vi "LaserExample.vi"() -> ()   [LabVIEW 2015]
panel:
  out "OK (Only RX Commands)":bool
  out "command received":bool
  out "Sended":bool
  in  "ENABLE LASER":bool
  out "Response":string
  out "error out":errorcluster
  in  "error in (no error)":errorcluster
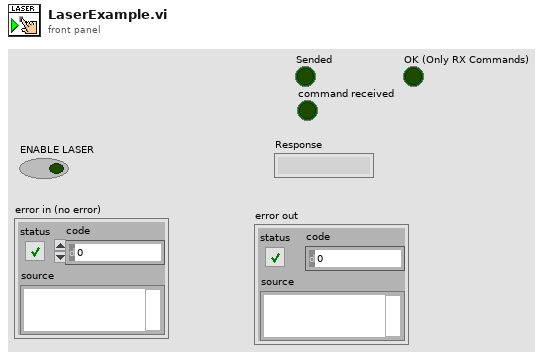
[diagram p1: front panel]
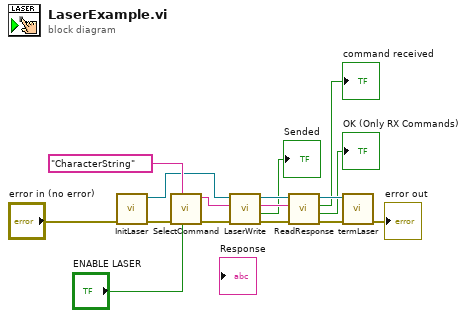
[diagram p0: block diagram]
diagram:
  n1 = call "InitLaser.vi"("error in (no error)"="error in (no error)") -> ("error out"=w6:errorcluster, "connection ID"=w5:refnum<k5>)  [unwired: 8 in]
  n2 = call "SelectCommand.vi"("ENABLE LASER"="ENABLE LASER", "SelectCommand"="CharacterString", "error in (no error)"=w6) -> ("error out"=w7:errorcluster, "Command"=w10:string)  [unwired: 7 in]
  n3 = call "LaserWrite.vi"("error in (no error)"=w7, "Command"=w10, "connection ID"=w5) -> ("error out"=w8:errorcluster, "Sended"=→"Sended":bool, "Command out"=w4:string, "connection ID out"=w9:refnum<k5>)  [unwired: 4 in]
  n4 = call "ReadResponse.vi"("error in (no error)"=w8, "Command"=w4, "connection ID"=w9) -> ("error out"=w13:errorcluster, "OK (Only RX Commands)"=→"OK (Only RX Commands)":bool, "command received"=→"command received":bool, "connection ID out"=w14:refnum<k5>)  [unwired: 5 in]
  n5 = call "termLaser.vi"("error in (no error)"=w13, "connection ID"=w14) -> ("error out"=→"error out":errorcluster)  [unwired: 9 in]
